vi "helper-snapshot-update.vi"(7 "Snapshot":T6[](array[typedef]) {"Dports" format="%08x"}, 9 "IO Map DI in":T5[](array[typedef]) {"ADDR" format="%04d"}, 10 "IO Map AI in":T1[](array[typedef]) {"ADDR" format="%04d"}, 11 "IO Map DO in":T4[](array[typedef]) {"ADDR" format="%04d"}) -> (1 "IO Map DI out":T5[](array[typedef]) {"ADDR" format="%04d"}, 2 "IO Map AI out":T1[](array[typedef]) {"ADDR" format="%04d"}, 3 "IO Map DO out":T4[](array[typedef]) {"ADDR" format="%04d"}, 4 "AI RAW":dbl[][](array[numeric]), 5 "AI":dbl[][](array[numeric]))   [LabVIEW 2024]
uses:
  controls/type-snapshot.ctl
  controls/type-io-map-di.ctl
  controls/type.address.ctl
  controls/enum.io.mode.ctl
  controls/type-io-map-do.ctl
  controls/type-io-map-ai.ctl
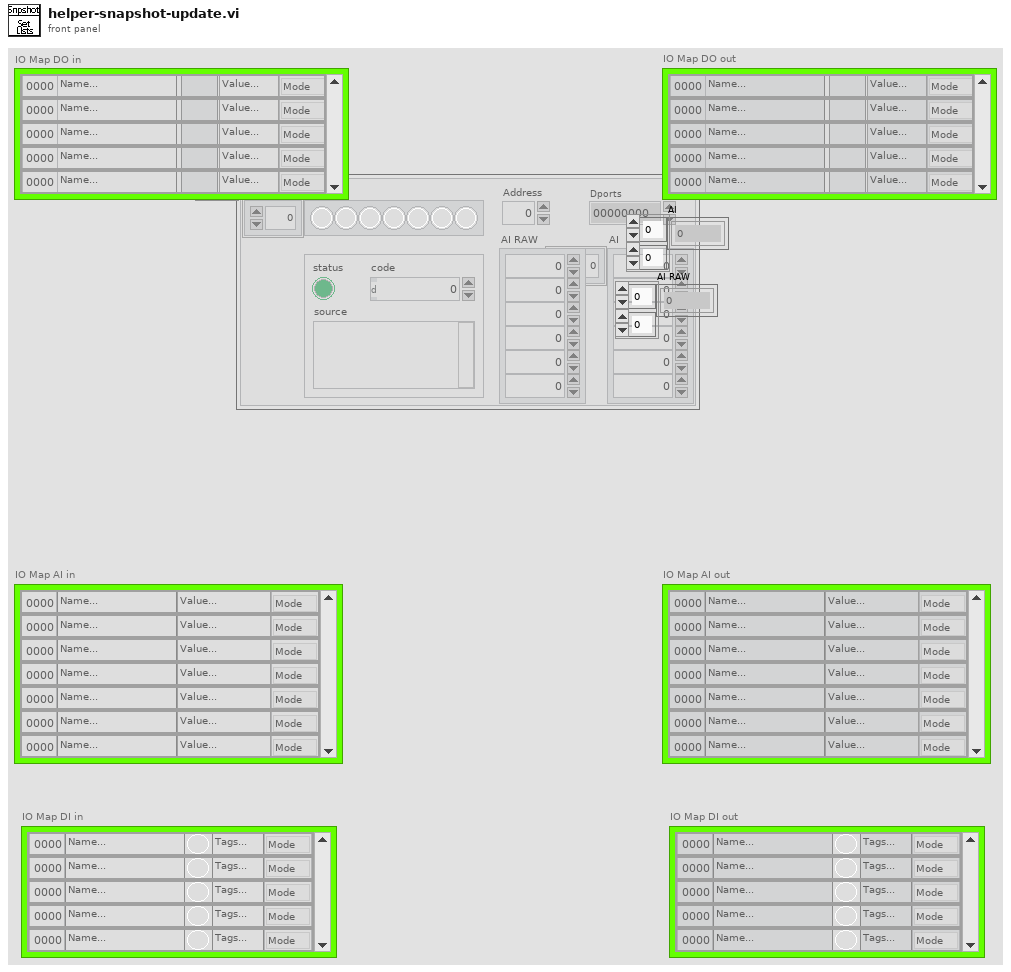
[diagram p1: front panel]
types:
  T1 = typedef "type-io-map-ai.ctl" = cluster{"ADDR":T2, "Label":string, "Mode":T3, "Value":string}
  T2 = typedef "type.address.ctl" = u16
  T3 = typedef "enum.io.mode.ctl" = enum16{"Mode", "RIO", "SIM"}
  T4 = typedef "type-io-map-do.ctl" = cluster{"ADDR":T2, "Label":string, "Mode":T3, "Value":string, "State":bool}
  T5 = typedef "type-io-map-di.ctl" = cluster{"ADDR":T2, "Label":string, "Mode":T3, "State":bool, "Value":string}
  T6 = typedef "type-snapshot.ctl" = cluster{"Address":u8, "DI":bool[], "status":errorcluster, "AI":dbl[], "Dports":u32, "AI RAW":dbl[]}
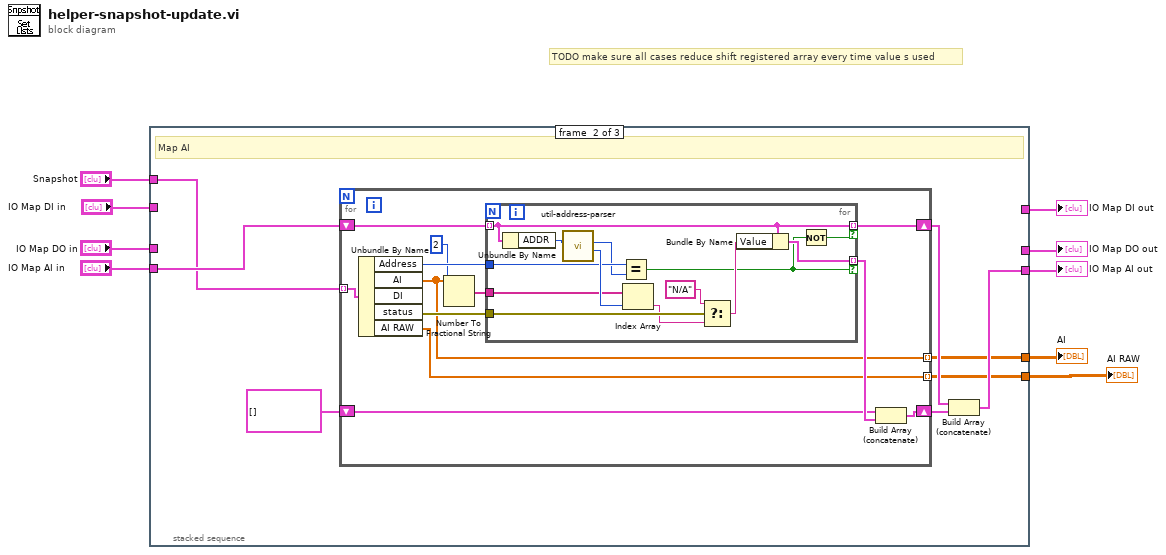
[diagram p0: block diagram]
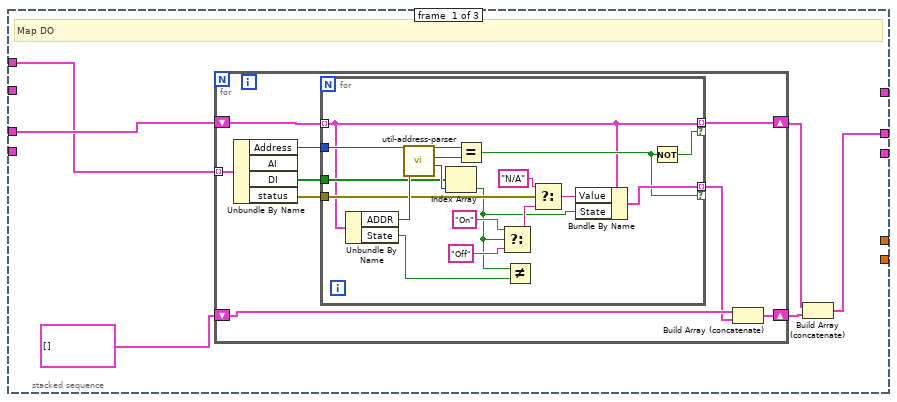
[diagram p2: hidden frame]
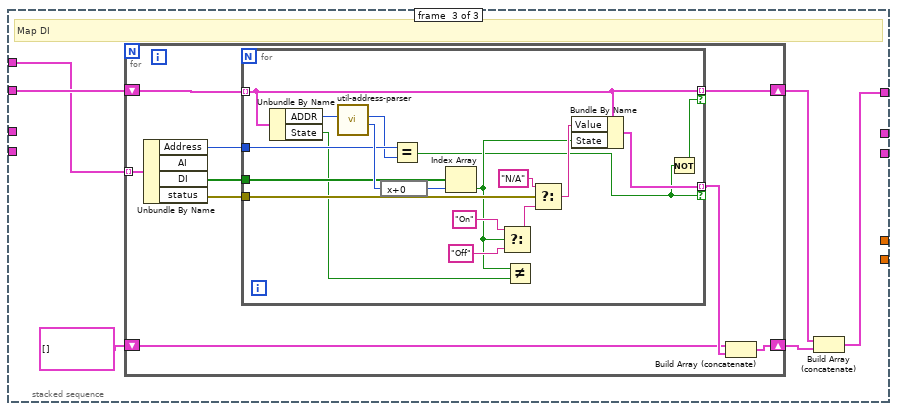
[diagram p3: hidden frame]
diagram:
  # "TODO make sure all cases reduce shift registered array every time value s used"
  n1 = stacked-sequence {
    tunnel: "IO Map DI in" -> [_ _ w79]
    tunnel: [_ _ w76] -> w5
    tunnel: "IO Map DO in" -> [w15 _ _]
    tunnel: [w11 _ _] -> w4
    tunnel: "IO Map AI in" -> [_ w49 _]
    tunnel: [_ w45 _] -> w3
    tunnel: "Snapshot" -> [w13 w48 w77]
    tunnel: [_ w43 _] -> w2
    tunnel: [_ w42 _] -> w1
    frame #0 {
      # "Map DO"
      n2 = for {
        tunnel: w13 -> [w24] mode=indexing
        shift-right: [w22] -> w10
        shift-left: w15 -> [w21]
        shift-right: [w17] -> w14
        shift-left: T4[] [] ("IO Map DO in 2") -> [w18]
        n3 = Unbundle By Name(w24) -> ("Address"=w23:u8, "DI"=w19:bool[], "status"=w20:errorcluster)  [unwired: 1 out]
        n4 = for {
          tunnel: w21 -> [w25] mode=indexing
          tunnel: [w25] -> w22 mode=indexing if=w26
          tunnel: w23 -> [w39]
          tunnel: w20 -> [w37]
          tunnel: w19 -> [w34]
          tunnel: [w28] -> w16 mode=indexing if=w27
          n5 = Unbundle By Name(w25) -> ("ADDR"=w41:T2, "State"=w29:bool)
          n6 = call "util-address-parser.vi"("ADDR 2"=w41) -> ("Channel"=w40:u8, "Address"=w38:u8)  [unwired: 9 in]
          n7 = Index Array(array=w34, index=w40) -> (element=w30:bool)
          n8 = Equal?(x=w39, y=w38) -> (x = y?=w27:bool)
          n9 = Select(t="On", s=w30, f="Off" ("t")) -> (s? t:f=w31:string)
          n10 = Not Equal?(x=w30, y=w29) -> ()  [unwired: 1 out]
          n11 = Select(t="N/A", s=w37, f=w31) -> (s? t:f=w36:string)
          n12 = Bundle By Name(cluster=w25, "Value"=w36, "State"=w30) -> (w28:T4)
          n13 = Not(x=w27) -> (.not. x?=w26:bool)
        }
        n14 = Build Array (concatenate)(w18, w16) -> (w17:T4[])
      }
      n15 = Build Array (concatenate)(w10, w14) -> (w11:T4[])
    }
    frame #1 {
      # "Map AI"
      n16 = for {
        tunnel: w48 -> [w61] mode=indexing
        shift-right: [w59] -> w44
        shift-left: w49 -> [w58]
        shift-right: [w52] -> w46
        shift-left: T1[] [] -> [w53]
        tunnel: [w51] -> w43 mode=indexing
        tunnel: [w50] -> w42 mode=indexing
        n17 = Unbundle By Name(w61) -> ("Address"=w60:u8, "AI"=w51:dbl[], "status"=w55:errorcluster, "AI RAW"=w50:dbl[])  [unwired: 1 out]
        n18 = Number To Fractional String(number=w51, precision (6)=i16 2) -> (F-format string=w57:string[])  [unwired: 2 in]
        n19 = for {
          tunnel: w58 -> [w62] mode=indexing
          tunnel: w57 -> [w72]
          tunnel: [w62] -> w59 mode=indexing if=w64
          tunnel: w60 -> [w71]
          tunnel: w55 -> [w69]
          tunnel: [w65] -> w54 mode=indexing if=w63
          n20 = Unbundle By Name(w62) -> ("ADDR"=w74:T2)
          n21 = call "util-address-parser.vi"("ADDR 2"=w74) -> ("Channel"=w73:u8, "Address"=w70:u8)  [unwired: 9 in]
          n22 = Equal?(x=w71, y=w70) -> (x = y?=w63:bool)
          n23 = Index Array(array=w72, index=w73) -> (element=w68:string)
          n24 = Select(t="N/A", s=w69, f=w68) -> (s? t:f=w67:string)
          n25 = Bundle By Name(cluster=w62, "Value"=w67) -> (w65:T1)
          n26 = Not(x=w63) -> (.not. x?=w64:bool)
        }
        n27 = Build Array (concatenate)(w53, w54) -> (w52:T1[])
      }
      n28 = Build Array (concatenate)(w44, w46) -> (w45:T1[])
    }
    frame #2 {
      # "Map DI"
      n29 = for {
        tunnel: w77 -> [w89] mode=indexing
        shift-right: [w87] -> w75
        shift-left: w79 -> [w86]
        shift-right: [w82] -> w78
        shift-left: T5[] [] -> [w81]
        n30 = Unbundle By Name(w89) -> ("Address"=w88:u8, "DI"=w84:bool[], "status"=w85:errorcluster)  [unwired: 1 out]
        n31 = for {
          tunnel: w86 -> [w90] mode=indexing
          tunnel: [w90] -> w87 mode=indexing if=w92
          tunnel: w88 -> [w105]
          tunnel: w85 -> [w103]
          tunnel: w84 -> [w100]
          tunnel: [w94] -> w83 mode=indexing if=w93
          n32 = Unbundle By Name(w90) -> ("ADDR"=w107:T2, "State"=w95:bool)
          n33 = call "util-address-parser.vi"("ADDR 2"=w107) -> ("Channel"=w106:u8, "Address"=w104:u8)  [unwired: 9 in]
          n34 = expression code="x+0"(w106) -> (w91:u8)
          n35 = Equal?(x=w105, y=w104) -> (x = y?=w93:bool)
          n36 = Index Array(array=w100, index=w91) -> (element=w96:bool)
          n37 = Select(t="On", s=w96, f="Off" ("t")) -> (s? t:f=w97:string)
          n38 = Not Equal?(x=w96, y=w95) -> ()  [unwired: 1 out]
          n39 = Select(t="N/A", s=w103, f=w97) -> (s? t:f=w102:string)
          n40 = Bundle By Name(cluster=w90, "Value"=w102, "State"=w96) -> (w94:T5)
          n41 = Not(x=w93) -> (.not. x?=w92:bool)
        }
        n42 = Build Array (concatenate)(w81, w83) -> (w82:T5[])
      }
      n43 = Build Array (concatenate)(w75, w78) -> (w76:T5[])
    }
  }
  "IO Map DI out" <- w5
  "IO Map DO out" <- w4
  "IO Map AI out" <- w3
  "AI" <- w2
  "AI RAW" <- w1
